vi "visa write.vi"(8 "error in (no error)":errorcluster, 9 "input":dbl format="%#.6g", 10 "delay before next writte (ms)":u32=500, 11 "VISA resource name":refnum<visa-resource-name>="COM4") -> (0 "error out":errorcluster, 3 "VISA resource name out":refnum<visa-resource-name>)   [LabVIEW 2015, in "485 comm Custom Device.lvlib"]
doc: "This example performs a serial port write and a serial port read. The parameters set for the serial port must match the parameters of the connected instrument or device. The VISA Configure Serial Port VI sets the configuration parameters. The front panel displays the controls used to configure the basic parameters, such as baud rate, data bits, and parity. The VI passes the VISA resource name to other VIs that perform operations on that VISA resource. The VISA Write function sends a command to the serial device and the VISA Read function returns data based on the command. The VISA Close function then closes the reference to the serial device. It is important to close the reference; otherwise, further communication through that port might not be possible."
uses:
  485 comm Custom Device.lvlib
panel:
  out "concatenated string":string
  out "bytes read":u32
  out "Response":string
  # "Overview: Demonstrates the use of the VISA functions to send a single command to a serial instrument and read a response.\nRequirements: NI-VISA Driver\nInstructions:\n1. Ensure the resource specified by the VISA resource name is a valid serial device.\n2. Run the VI.\n3. If your instrument recognizes the \"*IDN?\" command, it should return a Response."
  # "Note: For an example of how to perform continuous serial communication in a loop, open the Continuous Serial Write and Read.vi in the same folder as this example."
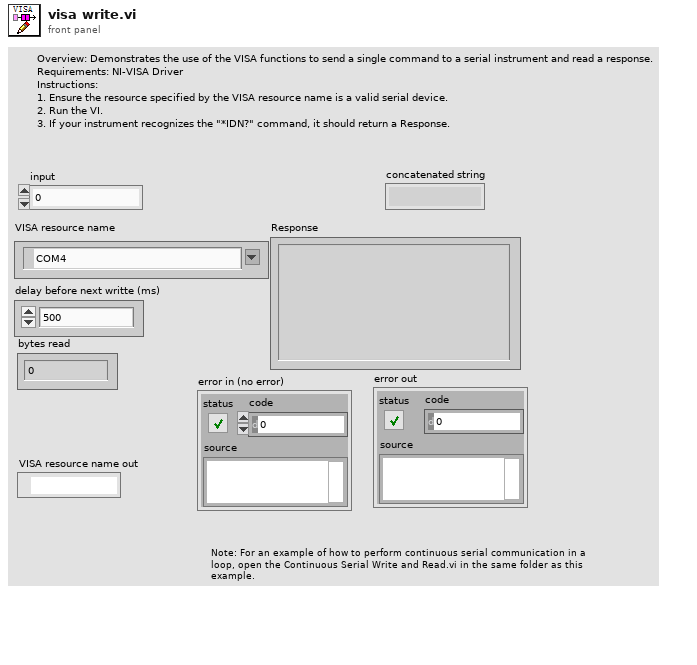
[diagram p1: front panel]
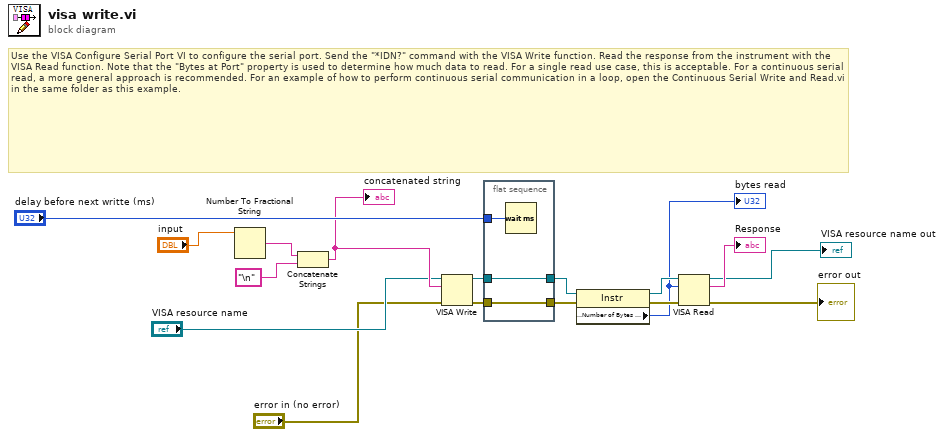
[diagram p0: block diagram]
diagram:
  # "Use the VISA Configure Serial Port VI to configure the serial port. Send the \"*IDN?\" command with the VISA Write function. Read the response from the instrument with the VISA Read function. Note that the \"Bytes at Port\" property is used to determine how much data to read. For a single read use case, this is acceptable. For a continuous serial read, a more general approach is recommended. For an example of how to perform continuous serial communication in a loop, open the Continuous Serial Write and Read.vi in the same folder as this example."
  n1 = Number To Fractional String(number="input") -> (F-format string=w8:string)  [unwired: 3 in]
  n2 = Concatenate Strings(w8, "\n" ("string")) -> (w6:string)
  "concatenated string" <- w6
  n3 = VISA Write(VISA resource name="VISA resource name", write buffer=w6, error in (no error)="error in (no error)") -> (VISA resource name out=w15:refnum<visa-resource-name>, error out=w17:errorcluster)  [unwired: 1 out]
  n4 = flat-sequence {
    tunnel: w17 -> [w19]
    tunnel: [w19] -> w16
    tunnel: w15 -> [w18]
    tunnel: [w18] -> w14
    tunnel: "delay before next writte (ms)" -> [w20]
    frame #0 {
      n5 = Wait (ms)(milliseconds to wait=w20) -> ()  [unwired: 1 out]
    }
  }
  n6 = property class="Instr"(reference=w14, error in=w16) -> (reference out=w12:refnum<visa-resource-name>, error out=w11:errorcluster, "Serial Settings:Number of Bytes at Serial Port"=w9:u32)
  "bytes read" <- w9
  n7 = VISA Read(VISA resource name=w12, byte count=w9, error in (no error)=w11) -> (VISA resource name out=→"VISA resource name out":refnum<visa-resource-name>, read buffer=→"Response":string, error out=→"error out":errorcluster)  [unwired: 1 out]
